vi "Logging Close.vi"(8 "error in (no error)":errorcluster, 11 "LoggingDevRef":T1) -> (0 "error out":errorcluster)   [LabVIEW 2012, in "femtoRoboLib.lvlib"]
doc: "Closes the reference to the counter you specify. Use this VI to close each counter reference that you open with the Open VI. If you do not stop a running counter with the Stop VI, closing the reference to the counter stops the counter.\n\nThis software is licensed. Open the labview\\readme\\WPI Robotics Library Open Source License.txt file for more information."
uses:
  femtoRoboLib.lvlib
  LoggingDevRef.ctl
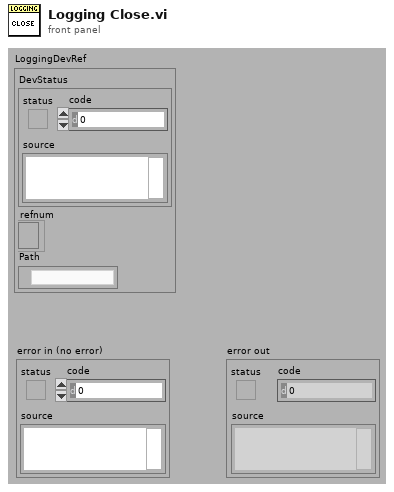
[diagram p1: front panel]
types:
  T1 = typedef "femtoRoboLib.lvlib/LoggingDevRef.ctl" = cluster{"DevStatus":errorcluster, "refnum":refnum<file>, "Path":path}
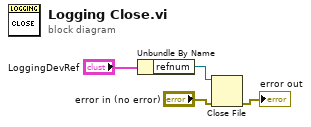
[diagram p0: block diagram]
diagram:
  n1 = Unbundle By Name("LoggingDevRef") -> ("refnum"=w3:refnum<file>)
  n2 = Close File(refnum=w3, error in="error in (no error)") -> (error out=→"error out":errorcluster)  [unwired: 1 out]
